vi "GOMDBTS2048 get Min Valid Wavelength.vi"(8 "error in (no error)":errorcluster, 11 "handle":i32) -> (0 "error out":errorcluster, 2 "function return":i32, 3 "value":dbl)   [LabVIEW 2015, in "GOMDBTS2048.lvlib"]
doc: "GOBTS2048DLL int __stdcall GOMDBTS2048_getMinValidWavelength(int handle, double* value);"
uses:
  GOMDBTS2048.lvlib
  runtime/GOMDBTS2048.dll
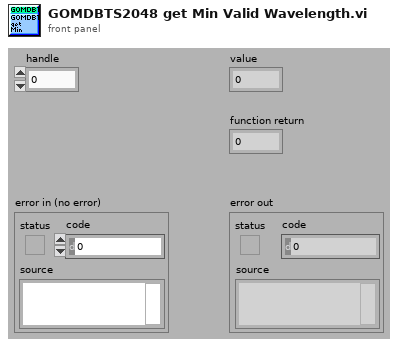
[diagram p1: front panel]
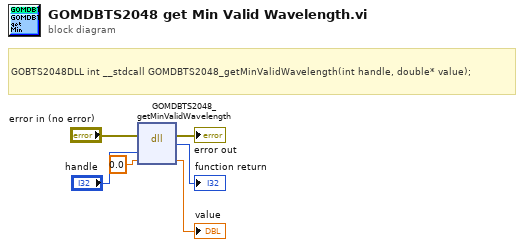
[diagram p0: block diagram]
diagram:
  # "GOBTS2048DLL int __stdcall GOMDBTS2048_getMinValidWavelength(int handle, double* value);"
  n1 = dll-call lib="C:/Users/rkoch/Documents/GO_Library/runtime/GOMDBTS2048.*" fn="GOMDBTS2048_getMinValidWavelength"(error in="error in (no error)", "handle"="handle", "value"=0.0) -> (error out=→"error out":errorcluster, →"function return":i32, "value"=→"value":dbl)  [unwired: 3 in, 1 out]
